vi "TTA_MATLAB_RFIC_Perform1TileATTTest.vi"(0 "Channel":string(combo), 1 "MXG VISA Resource In":refnum<visa-resource-name>, 2 "EXA VISA Resource":refnum<visa-resource-name>, 5 "Tx":string(combo), 7 "Freq_Cal_List":dbl, 9 "DigATT Values":T1, 11 "error in":errorcluster) -> (4 "Amp":dbl, 6 "Attenuation":dbl, 8 "Temp":dbl, 12 "MXG VISA Resource Out":refnum<visa-resource-name>, 13 "EXA VISA Resource Out":refnum<visa-resource-name>, 15 "error out":errorcluster)   [LabVIEW 2016]
panel:
  out "Tx#":i32
  out "CH#":i32
  out "IFFreq":dbl
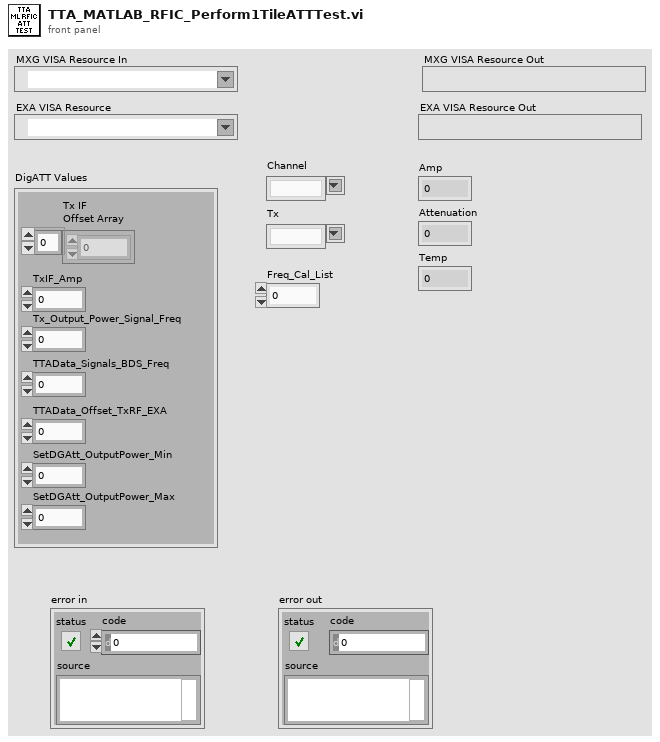
[diagram p1: front panel]
types:
  T1 = cluster{"Tx IF\nOffset Array":dbl[], "TxIF_Amp":dbl, "Tx_Output_Power_Signal_Freq":dbl, "TTAData_Signals_BDS_Freq":dbl, "TTAData_Offset_TxRF_EXA":dbl, "SetDGAtt_OutputPower_Min":dbl, "SetDGAtt_OutputPower_Max":dbl}
  T2 = enum16{"TX1", "TX2", "TX3", "TX4", "TXx3", "TXx4", "RX1", "RX2", "RX3", "RX4", "RXx3", "RXx4", "RFCal"}
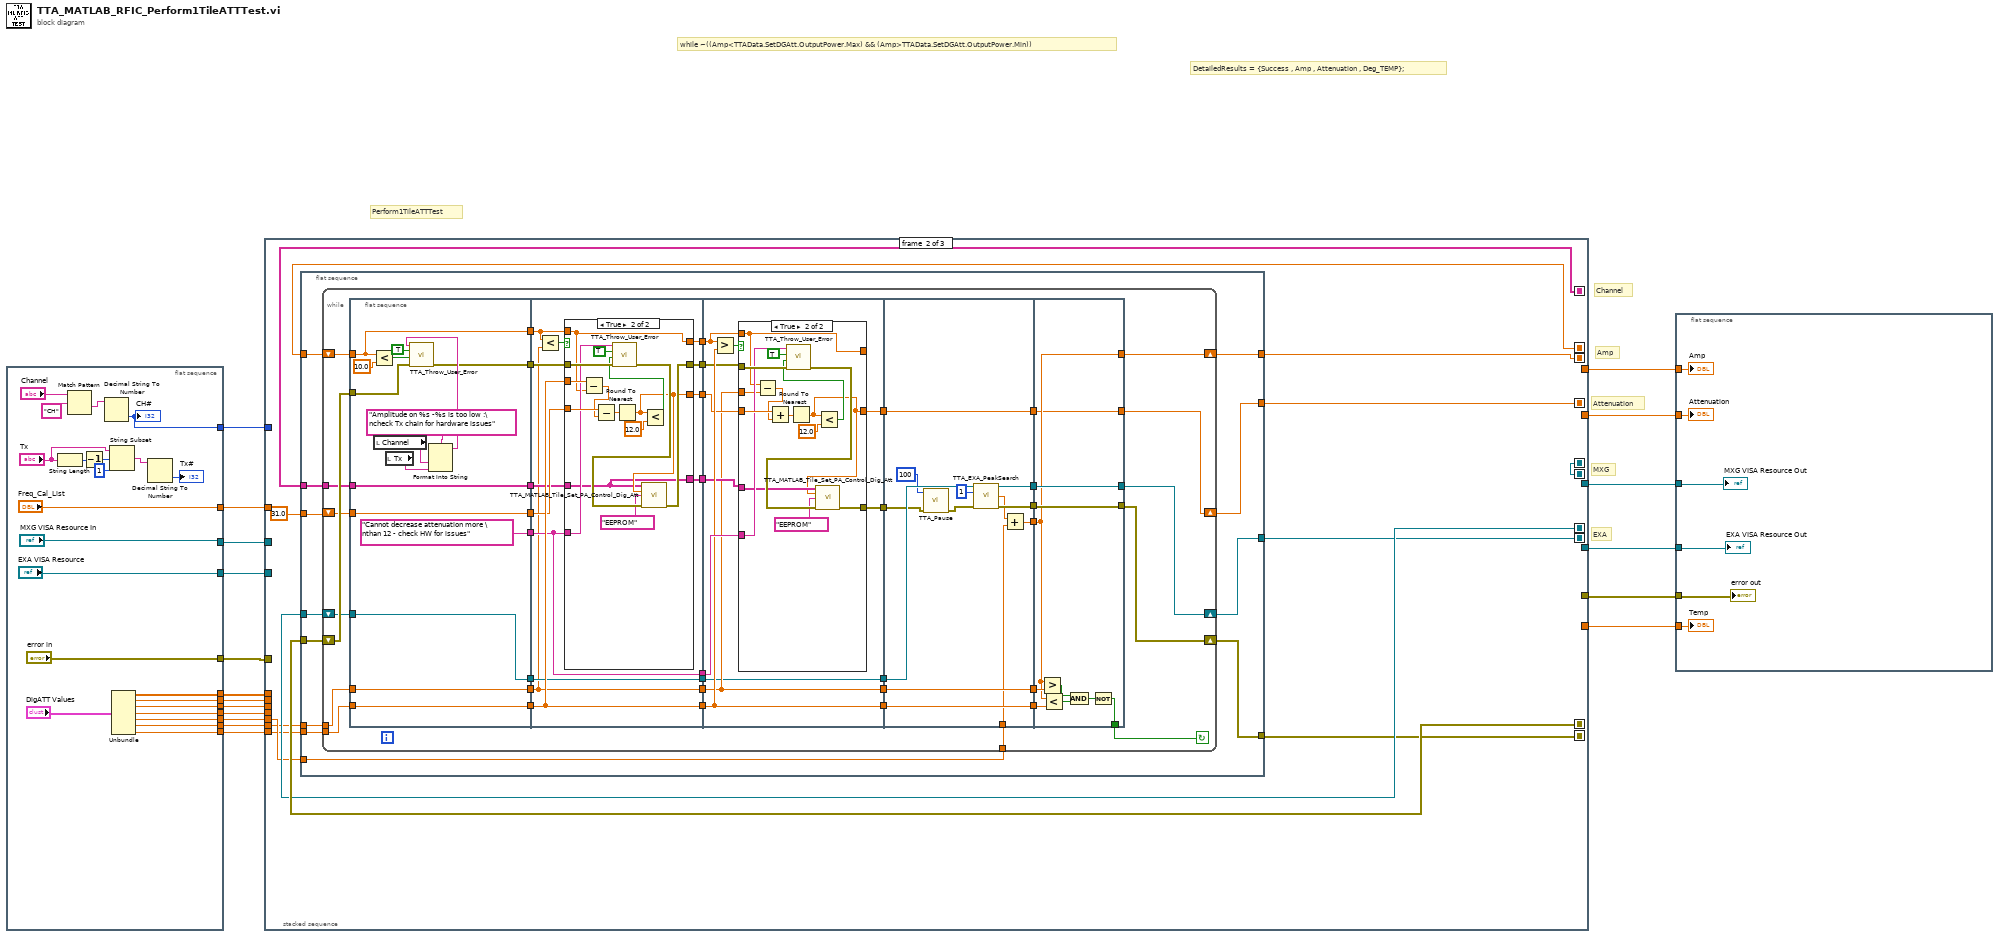
[diagram p0: block diagram]
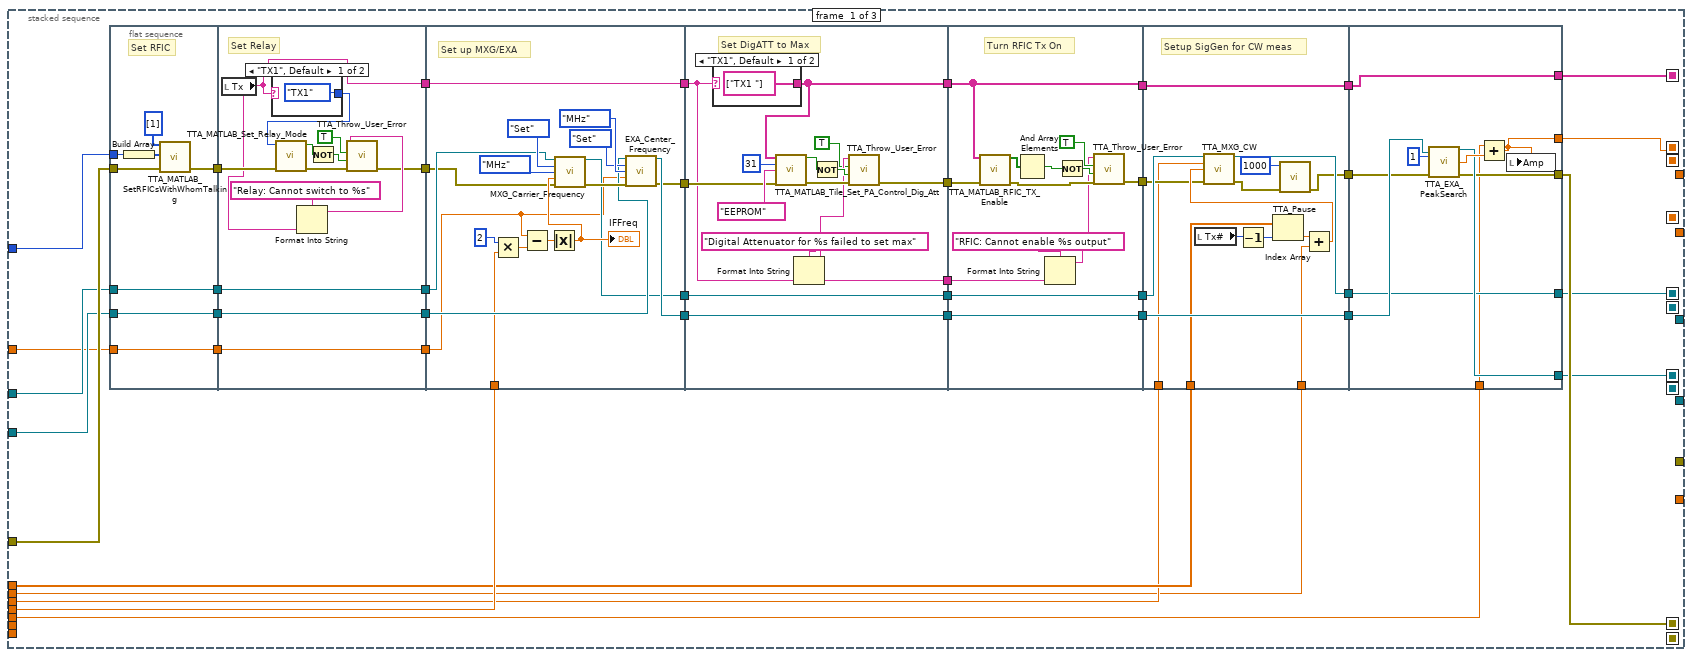
[diagram p2: hidden frame]
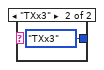
[diagram p3: hidden frame]
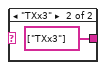
[diagram p4: hidden frame]
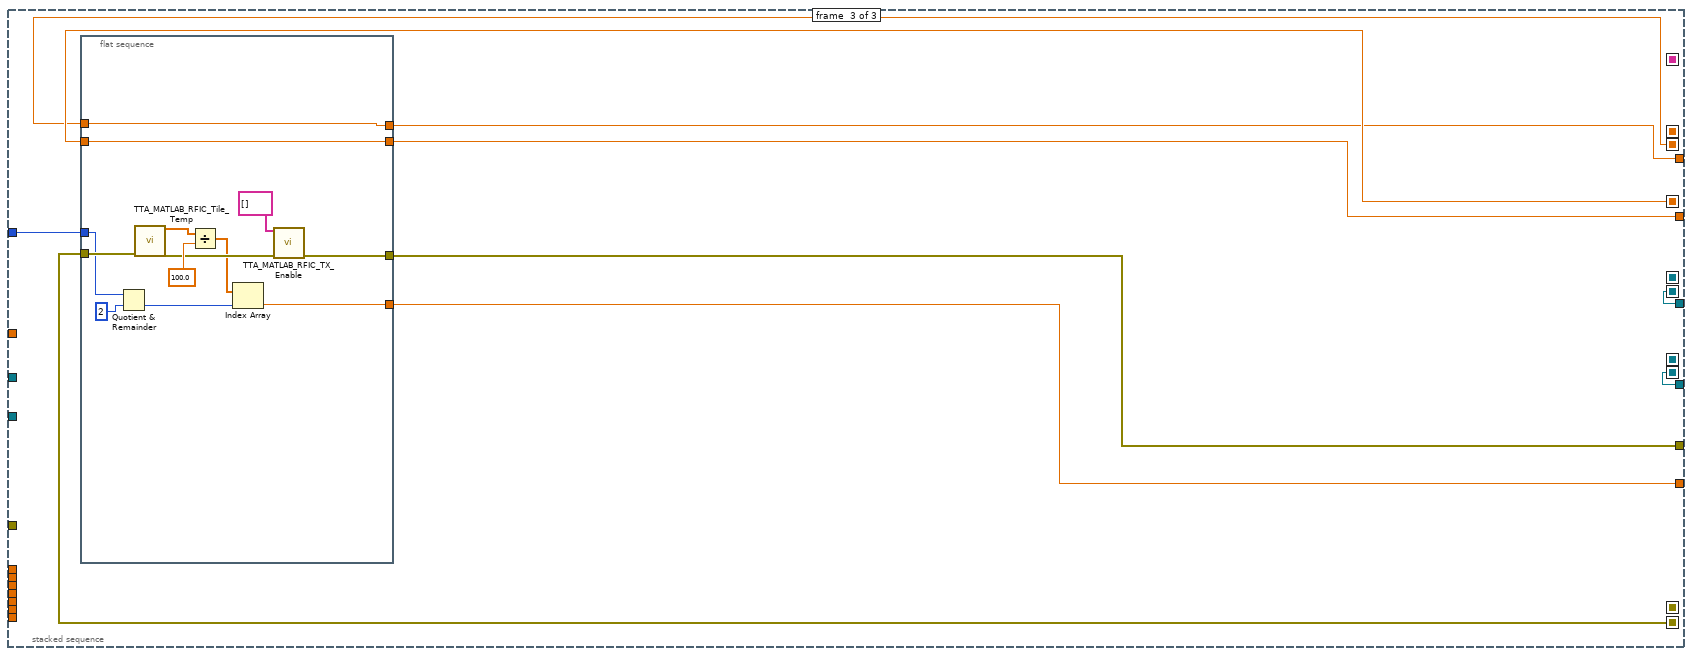
[diagram p7: hidden frame]
diagram:
  # "Attenuation"
  # "EXA"
  # "MXG"
  # "Channel"
  # "Amp"
  # "while ~((Amp<TTAData.SetDGAtt.OutputPower.Max) && (Amp>TTAData.SetDGAtt.OutputPower.Min))"
  # "DetailedResults = {Success , Amp , Attenuation , Deg_TEMP};"
  # "Perform1TileATTTest"
  n1 = flat-sequence {
    tunnel: ["error in"] -> w18
    tunnel: ["MXG VISA Resource In"] -> w16
    tunnel: ["EXA VISA Resource"] -> w15
    tunnel: [w34] -> w17
    tunnel: ["Freq_Cal_List"] -> w8
    tunnel: [w25] -> w7
    tunnel: [w24] -> w6
    tunnel: [w23] -> w5
    tunnel: [w22] -> w4
    tunnel: [w21] -> w3
    tunnel: [w20] -> w2
    tunnel: [w19] -> w1
    frame #0 {
      n2 = String Length(string="Tx") -> (length=w33:i32)
      n3 = Match Pattern(string="Channel", regular expression="CH") -> (after substring=w35:string)  [unwired: 1 in, 3 out]
      n4 = Decrement(x=w33) -> (x-1=w31:i32)
      n5 = Decimal String To Number(string=w35) -> (number=w34:i32)  [unwired: 2 in, 1 out]
      "CH#" <- w34
      n6 = String Subset(string="Tx", offset (0)=w31, length (rest)=1 ("length (rest)")) -> (substring=w29:string)
      n7 = Unbundle("DigATT Values") -> ("Tx IF\nOffset Array"=w24:dbl[], "TxIF_Amp"=w22:dbl, "Tx_Output_Power_Signal_Freq"=w23:dbl, "TTAData_Signals_BDS_Freq"=w25:dbl, "TTAData_Offset_TxRF_EXA"=w21:dbl, "SetDGAtt_OutputPower_Min"=w20:dbl, "SetDGAtt_OutputPower_Max"=w19:dbl)
      n8 = Decimal String To Number(string=w29) -> (number=→"Tx#":i32)  [unwired: 2 in, 1 out]
    }
  }
  n9 = stacked-sequence {
    seq-local: [w58 _ _] -> [_ w188 _]
    seq-local: [w55 _ _] -> [_ w183 _]
    seq-local: [w54 _ _] -> [_ w185 _]
    seq-local: [w53 _ _] -> [_ w189 _]
    seq-local: [w50 _ _] -> [_ w186 _]
    seq-local: [_ w184 _] -> [_ _ w351]
    seq-local: [_ w183 _] -> [_ _ w350]
    seq-local: [_ w182 _] -> [_ _ w349]
    seq-local: [_ w181 _] -> [_ _ w346]
    seq-local: [_ w180 _] -> [_ _ w347]
    tunnel: w18 -> [w81 _ _]
    tunnel: w17 -> [w80 _ w348]
    tunnel: w16 -> [w77 _ _]
    tunnel: w15 -> [w76 _ _]
    tunnel: [_ _ w351] -> w14
    tunnel: [_ _ w350] -> w13
    tunnel: [_ _ w345] -> w10
    tunnel: [_ _ w344] -> w11
    tunnel: [_ _ w343] -> w12
    tunnel: [_ _ w342] -> w9
    tunnel: w8 -> [w49 _ _]
    tunnel: w7 -> [w46 _ _]
    tunnel: w6 -> [w45 _ _]
    tunnel: w5 -> [w44 _ _]
    tunnel: w4 -> [w43 _ _]
    tunnel: w3 -> [w42 w179 _]
    tunnel: w2 -> [_ w178 _]
    tunnel: w1 -> [_ w177 _]
    frame #0 {
      n10 = flat-sequence {
        tunnel: w81 -> [w89]
        tunnel: w80 -> [w86]
        tunnel: [w85] -> w79
        tunnel: w77 -> [w84]
        tunnel: w76 -> [w83]
        tunnel: [w84] -> w75
        tunnel: [w83] -> w74
        tunnel: w49 -> [w82]
        tunnel: [w82] -> w48
        tunnel: w79 -> [w102]
        tunnel: [w94] -> w78
        tunnel: w75 -> [w93]
        tunnel: w74 -> [w92]
        tunnel: [w93] -> w73
        tunnel: [w92] -> w72
        tunnel: [w91] -> w67
        tunnel: w48 -> [w90]
        tunnel: [w90] -> w47
        tunnel: w78 -> [w109]
        tunnel: w73 -> [w113]
        tunnel: w72 -> [w112]
        tunnel: [w111] -> w71
        tunnel: [w110] -> w70
        tunnel: [w108] -> w69
        tunnel: [w107] -> w68
        tunnel: w67 -> [w107]
        tunnel: w47 -> [w106]
        tunnel: w46 -> [w105]
        tunnel: w71 -> [w123]
        tunnel: w70 -> [w124]
        tunnel: w69 -> [w134]
        tunnel: w68 -> [w125]
        tunnel: [w127] -> w66
        tunnel: [w126] -> w65
        tunnel: [w125] -> w64
        tunnel: [w124] -> w62
        tunnel: [w123] -> w61
        tunnel: w66 -> [w151]
        tunnel: w65 -> [w139]
        tunnel: w64 -> [w144]
        tunnel: [w142] -> w63
        tunnel: w62 -> [w141]
        tunnel: w61 -> [w140]
        tunnel: [w141] -> w60
        tunnel: [w140] -> w59
        tunnel: [w139] -> w52
        tunnel: w63 -> [w161]
        tunnel: w60 -> [w162]
        tunnel: w59 -> [w160]
        tunnel: [w160] -> w57
        tunnel: [w159] -> w56
        tunnel: w52 -> [w158]
        tunnel: [w158] -> w51
        tunnel: w45 -> [w157]
        tunnel: w44 -> [w156]
        tunnel: w43 -> [w155]
        tunnel: [w153] -> w41
        tunnel: [w174] -> w54
        tunnel: [w173] -> w58
        tunnel: w57 -> [w172]
        tunnel: w56 -> [w171]
        tunnel: [w171] -> w55
        tunnel: [w169] -> w53
        tunnel: w51 -> [w170]
        tunnel: [w170] -> w50
        tunnel: w42 -> [w168]
        tunnel: w41 -> [w167]
        frame #0 {
          # "Set RFIC"
          n11 = Build Array(w86) -> (w87:i32[])
          n12 = call "TTA_MATLAB_SetRFICsWithWhomTalking.vi"("Panel Array"=i32[] [1], "RFIC Array"=w87, "error in"=w89) -> ("error out"=w85:errorcluster)  [unwired: 12 in]
        }
        frame #1 {
          # "Set Relay"
          n13 = local read "Tx"() -> (w91:string)
          n14 = case shown="\"TX1\", Default" w91 {
            tunnel: [T2."TX1" ("Mode") T2."TXx3" ("Mode")] -> w101
            frame "TX1", Default {
            }
            frame "TXx3" {
            }
          }
          n15 = call "TTA_MATLAB_Set_Relay_Mode.vi"("error in"=w102, "Mode"=w101) -> ("error out"=w100:errorcluster, "Success"=w99:bool)  [unwired: 8 in]
          n16 = Format Into String(format string="Relay: Cannot switch to %s", w91) -> (resulting string=w95:string)  [unwired: 2 in, 1 out]
          n17 = Not(x=w99) -> (.not. x?=w98:bool)
          n18 = call "TTA_Throw_User_Error.vi"("error in"=w100, "Error?"=w98, "Stop Execution on Fail"=TRUE, "Error Message"=w95) -> ("error out"=w94:errorcluster)  [unwired: 7 in]
        }
        frame #2 {
          # "Set up MXG/EXA"
          n19 = Multiply(x=2, y=w105) -> (x*y=w115:dbl)
          n20 = Subtract(x=w106, y=w115) -> (x-y=w116:dbl)
          n21 = Absolute Value(x=w116) -> (abs(x)=w122:dbl)
          "IFFreq" <- w122
          n22 = call "MXG_Carrier_Frequency.vi"("VISA resource name"=w113, "Mode"=enum16{"Set", "Get"}."Set", "Units"=enum16{"Hz", "kHz", "MHz", "GHz"}."MHz", "Frequency"=w122, "error in"=w109) -> ("VISA resource name"=w110:refnum<visa-resource-name>, "error out"=w119:errorcluster)  [unwired: 8 in, 1 out]
          n23 = call "EXA_Center_Frequency.vi"("VISA resource name"=w112, "Mode"=enum16{"Set", "Get"}."Set", "Units"=enum16{"Hz", "kHz", "MHz", "GHz"}."MHz", "Frequency"=w106, "error in"=w119) -> ("VISA resource name"=w111:refnum<visa-resource-name>, "error out"=w108:errorcluster)  [unwired: 8 in, 1 out]
        }
        frame #3 {
          # "Set DigATT to Max"
          n24 = case shown="\"TX1\", Default" w125 {
            tunnel: [string[] ["TX1 "] ("Channels") string[] ["TXx3"] ("Channels")] -> w126
            frame "TX1", Default {
            }
            frame "TXx3" {
            }
          }
          n25 = call "TTA_MATLAB_Tile_Set_PA_Control_Dig_Att.vi"("Channels"=w126, "Attenuation (dB)"=31, "Mode"="EEPROM", "error in"=w134) -> ("Success"=w131:bool, "error out"=w133:errorcluster)  [unwired: 8 in, 2 out]
          n26 = Format Into String(format string="Digital Attenuator for %s failed to set max", w125) -> (resulting string=w129:string)  [unwired: 2 in, 1 out]
          n27 = Not(x=w131) -> (.not. x?=w132:bool)
          n28 = call "TTA_Throw_User_Error.vi"("error in"=w133, "Error?"=w132, "Stop Execution on Fail"=TRUE, "Error Message"=w129) -> ("error out"=w127:errorcluster)  [unwired: 7 in]
        }
        frame #4 {
          # "Turn RFIC Tx On"
          n29 = call "TTA_MATLAB_RFIC_TX_Enable.vi"("Channels"=w139, "error in"=w151) -> ("SuccessComm"=w150:bool[], "error out"=w146:errorcluster)  [unwired: 12 in]
          n30 = And Array Elements(Boolean array=w150) -> (logical AND=w147:bool)
          n31 = Format Into String(format string="RFIC: Cannot enable %s output", w144) -> (resulting string=w143:string)  [unwired: 2 in, 1 out]
          n32 = Not(x=w147) -> (.not. x?=w148:bool)
          n33 = call "TTA_Throw_User_Error.vi"("error in"=w146, "Error?"=w148, "Stop Execution on Fail"=TRUE, "Error Message"=w143) -> ("error out"=w142:errorcluster)  [unwired: 7 in]
        }
        frame #5 {
          # "Setup SigGen for CW meas"
          n34 = local read "Tx#"() -> (w165:i32)
          n35 = Decrement(x=w165) -> (x-1=w164:i32)
          n36 = Index Array(array=w157, index=w164) -> (element=w163:dbl)
          n37 = Add(x=w163, y=w155) -> (x+y=w166:dbl)
          n38 = call "TTA_MXG_CW.vi"("VISA resource In"=w162, "Frequency (MHz)"=w156, "Output Power\nLevel (dBm)"=w166, "error in"=w161) -> ("VISA resource Out"=w159:refnum<visa-resource-name>, "error out"=w154:errorcluster)  [unwired: 10 in]
          n39 = call "TTA_Pause.vi"("error in"=w154, "Pause (ms)"=u32 1000) -> ("error out"=w153:errorcluster)  [unwired: 9 in]
        }
        frame #6 {
          n40 = call "TTA_EXA_PeakSearch.vi"("VISA resource In"=w172, "Marker\nNumber"=1 ("Marker\nNumber"), "error in"=w167) -> ("VISA resource Out"=w174:refnum<visa-resource-name>, "Amplitude (dBm)"=w176:dbl, "error out"=w173:errorcluster)  [unwired: 9 in, 1 out]
          n41 = Add(x=w168, y=w176) -> (x+y=w169:dbl)
          n42 = local write "Amp"(w169) -> ()
        }
      }
    }
    frame #1 {
      n43 = flat-sequence {
        tunnel: w189 -> [w201]
        tunnel: w188 -> [w200]
        tunnel: 31.0 -> [w199]
        tunnel: w186 -> [w198]
        tunnel: w185 -> [w197]
        tunnel: [w196] -> w184
        tunnel: [w195] -> w182
        tunnel: [w194] -> w181
        tunnel: [w193] -> w180
        tunnel: w179 -> [w192]
        tunnel: w178 -> [w191]
        tunnel: w177 -> [w190]
        frame #0 {
          n44 = while {
            shift-right: [w208] -> w194
            shift-left: w201 -> [w236]
            shift-right: [w209] -> w195
            shift-left: w200 -> [w235]
            shift-right: [w205] -> w193
            shift-left: w199 -> [w232]
            tunnel: w198 -> [w229]
            shift-right: [w212] -> w196
            shift-left: w197 -> [w216]
            tunnel: w192 -> [w204]
            tunnel: w191 -> [w203]
            tunnel: w190 -> [w202]
            stop <- w241 continue-if-true
            n45 = flat-sequence {
              tunnel: [w243] -> w240
              tunnel: [w242] -> w239
              tunnel: w236 -> [w248]
              tunnel: w235 -> [w255]
              tunnel: [w249] -> w234
              tunnel: [w248] -> w233
              tunnel: w232 -> [w247]
              tunnel: [w247] -> w231
              tunnel: ["Cannot decrease attenuation more \nthan 12 - check HW for issues" ("Error Message")] -> w230
              tunnel: w229 -> [w245]
              tunnel: [w245] -> w228
              tunnel: [w244] -> w217
              tunnel: w216 -> [w244]
              tunnel: w203 -> [w243]
              tunnel: w202 -> [w242]
              tunnel: w240 -> [w258]
              tunnel: w239 -> [w268]
              tunnel: [w268] -> w238
              tunnel: [w258] -> w237
              tunnel: w234 -> [w269]
              tunnel: w233 -> [w264]
              tunnel: w231 -> [w267]
              tunnel: w230 -> [w265]
              tunnel: w228 -> [w266]
              tunnel: [w265] -> w227
              tunnel: [w263] -> w226
              tunnel: [w262] -> w225
              tunnel: [w261] -> w224
              tunnel: [w260] -> w223
              tunnel: w217 -> [w259]
              tunnel: [w259] -> w215
              tunnel: [w298] -> w222
              tunnel: w238 -> [w298]
              tunnel: [w294] -> w220
              tunnel: w237 -> [w294]
              tunnel: w227 -> [w300]
              tunnel: w226 -> [w297]
              tunnel: w225 -> [w296]
              tunnel: w224 -> [w295]
              tunnel: w223 -> [w293]
              tunnel: [w292] -> w218
              tunnel: w215 -> [w291]
              tunnel: [w291] -> w214
              tunnel: [w290] -> w206
              tunnel: w222 -> [w331]
              tunnel: [w331] -> w221
              tunnel: w220 -> [w330]
              tunnel: [w330] -> w219
              tunnel: w218 -> [w319]
              tunnel: w214 -> [w328]
              tunnel: [w327] -> w213
              tunnel: [w326] -> w211
              tunnel: [w324] -> w210
              tunnel: [w323] -> w207
              tunnel: w206 -> [w323]
              tunnel: w204 -> [w322]
              tunnel: [w338] -> w241
              tunnel: w221 -> [w337]
              tunnel: w219 -> [w336]
              tunnel: w213 -> [w335]
              tunnel: [w335] -> w212
              tunnel: w211 -> [w334]
              tunnel: w210 -> [w333]
              tunnel: [w334] -> w209
              tunnel: [w333] -> w208
              tunnel: w207 -> [w332]
              tunnel: [w332] -> w205
              frame #0 {
                n46 = Less?(x=w248, y=10.0) -> (x < y?=w256:bool)
                n47 = local read "Channel"() -> (w253:string)
                n48 = local read "Tx"() -> (w252:string)
                n49 = Format Into String(format string="Amplitude on %s -%s is too low :\ncheck Tx chain for hardware issues" ("Error Message"), w253, w252) -> (resulting string=w251:string)  [unwired: 2 in, 1 out]
                n50 = call "TTA_Throw_User_Error.vi"("error in"=w255, "Error?"=w256, "Stop Execution on Fail"=TRUE, "Error Message"=w251) -> ("error out"=w249:errorcluster)  [unwired: 7 in]
              }
              frame #1 {
                n51 = Less?(x=w264, y=w258) -> (x < y?=w270:bool)
                n52 = case shown="True" w270 {
                  tunnel: w269 -> [w274 w284]
                  tunnel: w268 -> [_ w289]
                  tunnel: w264 -> [w271 w275]
                  tunnel: w267 -> [w273 w288]
                  tunnel: w265 -> [_ w283]
                  tunnel: w266 -> [w272 w276]
                  tunnel: [w274 w278] -> w263
                  tunnel: [w273 w277] -> w262
                  tunnel: [w272 w276] -> w261
                  tunnel: [w271 w275] -> w260
                  frame False {
                  }
                  frame True {
                    n53 = Subtract(x=w289, y=w275) -> (x-y=w287:dbl)
                    n54 = Subtract(x=w288, y=w287) -> (x-y=w286:dbl)
                    n55 = Round To Nearest(number=w286) -> (nearest integer value=w277:dbl)
                    n56 = Less?(x=w277, y=12.0) -> (x < y?=w282:bool)
                    n57 = call "TTA_Throw_User_Error.vi"("error in"=w284, "Error?"=w282, "Stop Execution on Fail"=TRUE, "Error Message"=w283) -> ("error out"=w280:errorcluster)  [unwired: 7 in]
                    n58 = call "TTA_MATLAB_Tile_Set_PA_Control_Dig_Att.vi"("Channels"=w276, "Attenuation (dB)"=w277, "Mode"="EEPROM", "error in"=w280) -> ("error out"=w278:errorcluster)  [unwired: 8 in, 3 out]
                  }
                }
              }
              frame #2 {
                n59 = Greater?(x=w293, y=w298) -> (0:w299:bool)
                n60 = case shown="True" w299 {
                  tunnel: w297 -> [w301 w314]
                  tunnel: w293 -> [w302 w306]
                  tunnel: w296 -> [w303 w318]
                  tunnel: w300 -> [_ w313]
                  tunnel: w295 -> [_ w309]
                  tunnel: w294 -> [_ w307]
                  tunnel: [w303 w305] -> w290
                  tunnel: [w302 w306] -> _
                  tunnel: [w301 w304] -> w292
                  frame False {
                  }
                  frame True {
                    n61 = Subtract(x=w306, y=w307) -> (x-y=w317:dbl)
                    n62 = Add(x=w318, y=w317) -> (x+y=w316:dbl)
                    n63 = Round To Nearest(number=w316) -> (nearest integer value=w305:dbl)
                    n64 = Less?(x=w305, y=12.0) -> (x < y?=w312:bool)
                    n65 = call "TTA_Throw_User_Error.vi"("error in"=w314, "Error?"=w312, "Stop Execution on Fail"=TRUE, "Error Message"=w313) -> ("error out"=w310:errorcluster)  [unwired: 7 in]
                    n66 = call "TTA_MATLAB_Tile_Set_PA_Control_Dig_Att.vi"("Channels"=w309, "Attenuation (dB)"=w305, "Mode"="EEPROM", "error in"=w310) -> ("error out"=w304:errorcluster)  [unwired: 8 in, 3 out]
                  }
                }
              }
              frame #3 {
                n67 = call "TTA_Pause.vi"("error in"=w319, "Pause (ms)"=u32 100) -> ("error out"=w321:errorcluster)  [unwired: 9 in]
                n68 = call "TTA_EXA_PeakSearch.vi"("VISA resource In"=w328, "Marker\nNumber"=1 ("Marker\nNumber"), "error in"=w321) -> ("VISA resource Out"=w327:refnum<visa-resource-name>, "Amplitude (dBm)"=w325:dbl, "error out"=w326:errorcluster)  [unwired: 9 in, 1 out]
                n69 = Add(x=w325, y=w322) -> (x+y=w324:dbl)
              }
              frame #4 {
                n70 = Greater?(x=w333, y=w336) -> (0:w341:bool)
                n71 = Less?(x=w333, y=w337) -> (x < y?=w340:bool)
                n72 = And(x=w341, y=w340) -> (x .and. y?=w339:bool)
                n73 = Not(x=w339) -> (.not. x?=w338:bool)
              }
            }
          }
        }
      }
    }
    frame #2 {
      n74 = flat-sequence {
        tunnel: w349 -> [w361]
        tunnel: w348 -> [w358]
        tunnel: w347 -> [w354]
        tunnel: w346 -> [w355]
        tunnel: [w355] -> w345
        tunnel: [w354] -> w344
        tunnel: [w353] -> w343
        tunnel: [w352] -> w342
        frame #0 {
          n75 = Quotient & Remainder(x=w358, y=2) -> (floor(x/y)=w356:i32)  [unwired: 1 out]
          n76 = call "TTA_MATLAB_RFIC_Tile_Temp.vi"("error in"=w361) -> ("Results"=w362:dbl[], "error out"=w360:errorcluster)  [unwired: 11 in, 2 out]
          n77 = Divide(x=w362, y=100.0) -> (x/y=w359:dbl[])
          n78 = Index Array(array=w359, index=w356) -> (element=w353:dbl)
          n79 = call "TTA_MATLAB_RFIC_TX_Enable.vi"("Channels"=string[] [], "error in"=w360) -> ("error out"=w352:errorcluster)  [unwired: 12 in, 1 out]
        }
      }
    }
  }
  n80 = flat-sequence {
    tunnel: w14 -> [w370]
    tunnel: w13 -> [w369]
    tunnel: w12 -> [w368]
    tunnel: w11 -> [w367]
    tunnel: w10 -> [w366]
    tunnel: w9 -> [w365]
    frame #0 {
      "error out" <- w365
      "MXG VISA Resource Out" <- w369
      "EXA VISA Resource Out" <- w370
      "Temp" <- w368
      "Attenuation" <- w367
      "Amp" <- w366
    }
  }
